vi "Sti_Switch.vi"(9 "Integer32":i32, 11 "自定义浮点32":sgl) -> (1 "20B_StrOut":string)   [LabVIEW 2020]
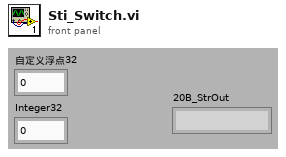
[diagram p1: front panel]
types:
  T1 = enum16{"big-endian, network order", "native, host order", "little-endian"}
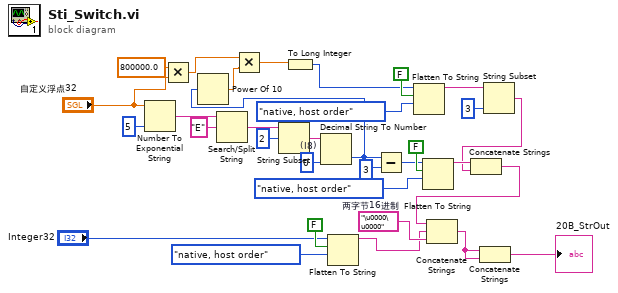
[diagram p0: block diagram]
diagram:
  w5 = "\u0000\u0000"  # 两字节16进制
  w25 = i8 0  # (I8)
  n1 = Number To Exponential String(number="自定义浮点32", precision (6)=i16 5 ("精度(6)")) -> (E-format string=w24:string)  [unwired: 2 in]
  n2 = Multiply(x=sgl 800000.0, y="自定义浮点32") -> (x*y=w11:sgl)
  n3 = Search/Split String(string=w24, search string/char (-)="E" ("搜索字符串/字符(-)")) -> (match + rest of string=w28:string)  [unwired: 1 in, 2 out]
  n4 = String Subset(string=w28, offset (0)=2 ("偏移量(0)")) -> (substring=w26:string)  [unwired: 1 in]
  n5 = Decimal String To Number(string=w26, default (0L)=w25) -> (number=w6:i8)  [unwired: 1 in, 1 out]
  n6 = Power Of 10(x=w6) -> (10^x=w10:dbl)
  n7 = Multiply(x=w11, y=w10) -> (x*y=w8:dbl)
  n8 = To Long Integer(number=w8) -> (32bit integer=w7:i32)
  n9 = Flatten To String(anything="Integer32", prepend array or string size? (T)=FALSE ("预置数组或字符串大小？(T)"), byte order (0:big-endian, network order)=T1."native, host order" ("字节顺序(0:big-endian, network order)")) -> (data string=w4:string)  [unwired: 1 in, 2 out]
  n10 = Subtract(x=w6, y=i8 3) -> (x-y=w9:i8)
  n11 = Flatten To String(anything=w7, prepend array or string size? (T)=FALSE ("预置数组或字符串大小？(T)"), byte order (0:big-endian, network order)=T1."native, host order" ("字节顺序(0:big-endian, network order)")) -> (data string=w19:string)  [unwired: 1 in, 2 out]
  n12 = Flatten To String(anything=w9, prepend array or string size? (T)=FALSE ("预置数组或字符串大小？(T)"), byte order (0:big-endian, network order)=T1."native, host order" ("字节顺序(0:big-endian, network order)")) -> (data string=w17:string)  [unwired: 1 in, 2 out]
  n13 = String Subset(string=w19, length (rest)=3 ("长度（剩余）")) -> (substring=w16:string)  [unwired: 1 in]
  n14 = Concatenate Strings(w17, w16) -> (w15:string)
  n15 = Concatenate Strings(w15, w4, w5) -> (w14:string)
  n16 = Concatenate Strings(w14, w14) -> (→"20B_StrOut":string)
